vi "滑移力曲线.vi"() -> ()   [LabVIEW 2020]
uses:
  Global_Variable/Global.vi
  Global_Variable/A131258.vi
panel:
  in  "拉装电缸压力":sgl
  in  "拉装电缸位移":sgl
  out "XY图":cluster{dbl[], dbl[]}[](graph)
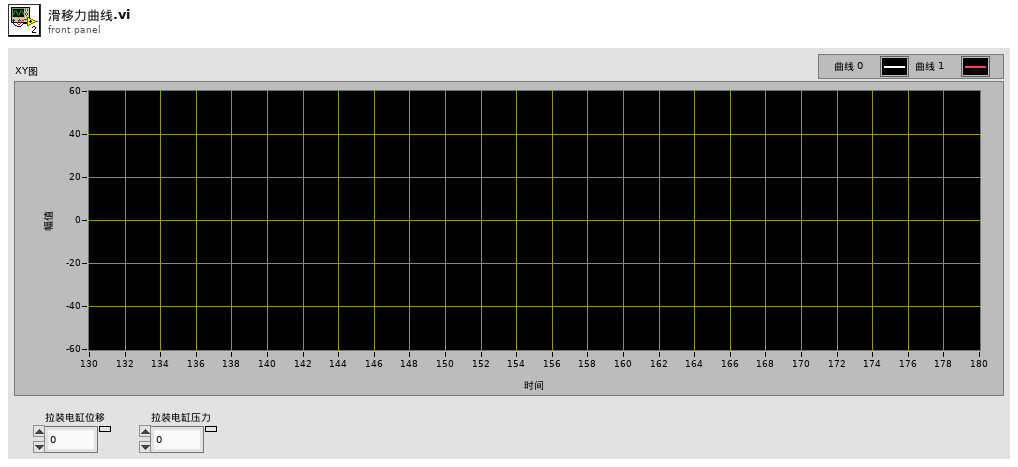
[diagram p1: front panel]
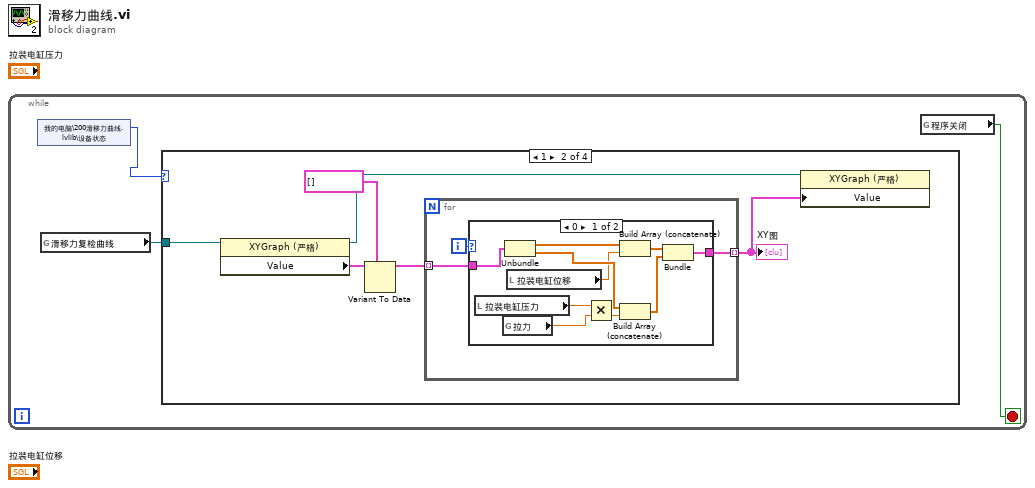
[diagram p0: block diagram]
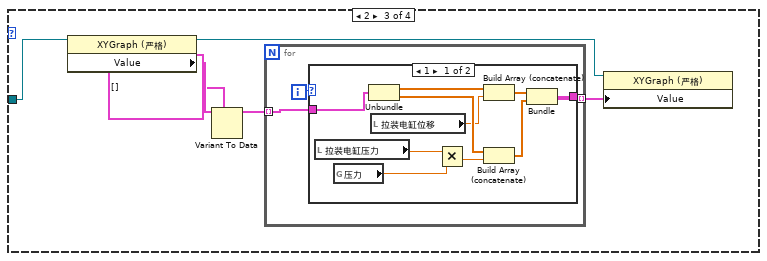
[diagram p4: hidden frame]
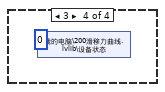
[diagram p6: hidden frame]
diagram:
  n1 = while {
    stop <- w3 stop-if-true
    n2 = shared-variable "我的电脑\\200滑移力曲线.lvlib\\设备状态"() -> (w1:u16)  [unwired: 1 in, 1 out]
    n3 = global read "Global.vi" "滑移力复检曲线"() -> (w2:refnum<vi>)
    n4 = case shown="1" w1 {
      tunnel: w2 -> [_ w9 w29 _]
      frame 0, Default {
      }
      frame 1 {
        n5 = property class="XYGraph (严格)"(reference=w9) -> (reference out=w5:refnum<vi>, "Value"=w8:cluster{dbl[], dbl[]}[])  [unwired: 1 in, 1 out]
        n6 = Variant To Data(type=cluster{dbl[], dbl[]}[] [], Variant=w8) -> (data=w6:cluster{dbl[], dbl[]}[])  [unwired: 1 in, 1 out]
        n7 = for {
          tunnel: w6 -> [w11] mode=indexing
          tunnel: [w10] -> w4 mode=indexing
          i -> [w12]
          n8 = case shown="0" w12 {
            tunnel: w11 -> [w22 w23]
            tunnel: [w17 w23] -> w10
            frame 0 {
              n9 = local read "拉装电缸压力"() -> (w14:sgl)
              n10 = global read "A131258.vi" "拉力"() -> (w13:dbl)
              n11 = Unbundle(w22) -> (w21:dbl[], w20:dbl[])
              n12 = local read "拉装电缸位移"() -> (w16:sgl)
              n13 = Multiply(x=w14, y=w13) -> (x*y=w15:dbl)
              n14 = Build Array (concatenate)(w21, w16) -> (w19:dbl[])
              n15 = Build Array (concatenate)(w20, w15) -> (w18:dbl[])
              n16 = Bundle(w19, w18) -> (w17:cluster{dbl[], dbl[]})  [unwired: 1 in]
            }
            frame Default {
            }
          }
        }
        "XY图" <- w4
        n17 = property class="XYGraph (严格)"(reference=w5, "Value"=w4) -> ()  [unwired: 1 in, 2 out]
      }
      frame 2 {
        n18 = property class="XYGraph (严格)"(reference=w29) -> (reference out=w25:refnum<vi>, "Value"=w28:cluster{dbl[], dbl[]}[])  [unwired: 1 in, 1 out]
        n19 = Variant To Data(type=cluster{dbl[], dbl[]}[] [] ("滑移力复检曲线"), Variant=w28) -> (data=w26:cluster{dbl[], dbl[]}[])  [unwired: 1 in, 1 out]
        n20 = for {
          tunnel: w26 -> [w31] mode=indexing
          tunnel: [w30] -> w24 mode=indexing
          i -> [w32]
          n21 = case shown="1" w32 {
            tunnel: w31 -> [w42 w43]
            tunnel: [w37 w43] -> w30
            frame 1 {
              n22 = local read "拉装电缸压力"() -> (w34:sgl)
              n23 = global read "A131258.vi" "压力"() -> (w33:dbl)
              n24 = Unbundle(w42) -> (w41:dbl[], w40:dbl[])
              n25 = local read "拉装电缸位移"() -> (w36:sgl)
              n26 = Multiply(x=w34, y=w33) -> (x*y=w35:dbl)
              n27 = Build Array (concatenate)(w41, w36) -> (w39:dbl[])
              n28 = Build Array (concatenate)(w40, w35) -> (w38:dbl[])
              n29 = Bundle(w39, w38) -> (w37:cluster{dbl[], dbl[]})  [unwired: 1 in]
            }
            frame Default {
            }
          }
        }
        n30 = property class="XYGraph (严格)"(reference=w25, "Value"=w24) -> ()  [unwired: 1 in, 2 out]
      }
      frame 3 {
        n31 = shared-variable "我的电脑\\200滑移力曲线.lvlib\\设备状态"(u16 0 ("设备状态")) -> ()  [unwired: 1 in, 1 out]
      }
    }
    n32 = global read "Global.vi" "程序关闭"() -> (w3:bool)
  }
